vi "PPS Measure.vi"(8 "error in (no error)":errorcluster, 11 "IT-M6018C in":refnum<class "IT-M6018C.lvclass">) -> (0 "error out":errorcluster, 1 "Actual Current Limit (A)":dbl format="%.2f", 2 "Actual Voltage Level (V)":dbl format="%.2f", 3 "IT-M6018C out":refnum<class "IT-M6018C.lvclass">)   [LabVIEW 2023, in "HardwareAbstractionLayer_LVOOP.lvlib" / "IT-M6018C.lvclass"]
uses:
  IT-M6018C.lvclass
  IT-M6018C.lvclass/IT-M6018C.ctl
  <instrlib>/IT6000C/IT6000C.lvlib
  PowerSupply.lvclass
  <vilib>/Instr/_visa.llb/VISA Flush IO Buffer Mask.ctl
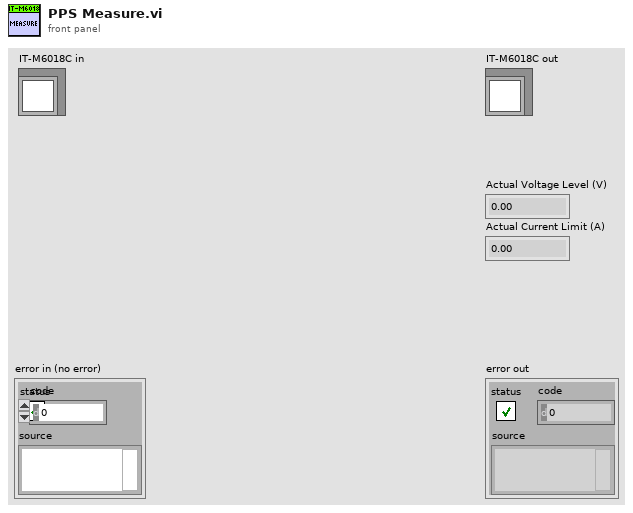
[diagram p1: front panel]
types:
  T1 = typedef "VISA Flush IO Buffer Mask.ctl" = u16
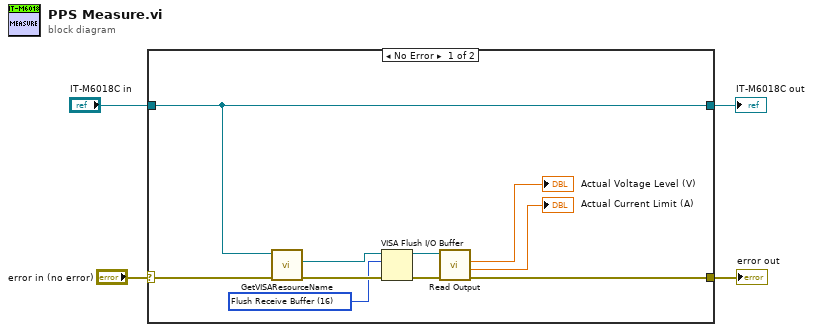
[diagram p0: block diagram]
diagram:
  n1 = case shown="No Error" "error in (no error)" {
    selector: "error in (no error)" -> [w11 w16]
    tunnel: [w12 w16] -> w3
    tunnel: "IT-M6018C in" -> [w10 w15]
    tunnel: [w10 w15] -> w1
    frame No Error {
      w5 = T1 16 items=["Flush Receive Buffer"=16, "Write Transmit Buffer to Device"=32, "Flush Receive Buffer (No I/O)"=64, "Flush Transmit Buffer"=128] ("Mask")
      n2 = call "GetVISAResourceName.vi"("error in (no error)"=w11, "object in"=w10) -> ("error out"=w6:errorcluster, "VISA resource name"=w9:refnum<visa-resource-name>)  [unwired: 7 in, 1 out]
      n3 = VISA Flush I/O Buffer(VISA resource name=w9, mask (16)=w5, error in (no error)=w6) -> (VISA resource name out=w8:refnum<visa-resource-name>, error out=w7:errorcluster)
      n4 = call <instrlib>:"Read Output.vi"("error in (no error)"=w7, "VISA resource name"=w8) -> ("error out"=w12:errorcluster, "Actual Current Level (A)"=→"Actual Current Limit (A)":dbl, "Actual Voltage Level (V)"=→"Actual Voltage Level (V)":dbl)  [unwired: 6 in, 1 out]
    }
    frame Error {
    }
  }
  "error out" <- w3
  "IT-M6018C out" <- w1
